vi "Check wait.vi"(11 "Trigger":refnum<vi>) -> (3 "Wait done?":bool)   [LabVIEW 2016]
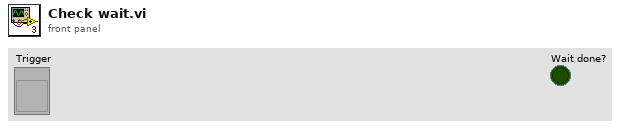
[diagram p1: front panel]
types:
  T1 = typedef "Test settings.ctl" = cluster{"Speed (mm/s)":dbl, "Position limit":bool, "Position limit (mm)":dbl, "Load limit":bool, "Load limit (N)":dbl, "No. of repeats":u16, "Test identifier":string, "Time wait":bool, "Wait time (s)":dbl, "Trigger wait":bool, "Send trigger":bool, "Test notes":string, "Snap intervals":bool, "Time interval (s)":dbl}
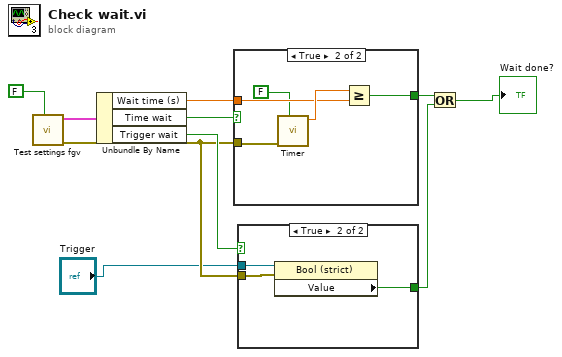
[diagram p0: block diagram]
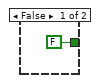
[diagram p2: hidden frame]
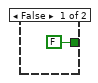
[diagram p3: hidden frame]
diagram:
  n1 = call "Test settings fgv.vi"("Set?"=FALSE) -> ("error out"=w2:errorcluster, "Test settings out"=w9:T1)  [unwired: 8 in, 1 out]
  n2 = Unbundle By Name(w9) -> ("Wait time (s)"=w7:dbl, "Time wait"=w8:bool, "Trigger wait"=w6:bool)
  n3 = case shown="True" w8 {
    tunnel: w2 -> [_ w16]
    tunnel: w7 -> [_ w14]
    tunnel: [FALSE w13] -> w5
    frame False {
    }
    frame True {
      n4 = call "Timer.vi"("Reset"=FALSE, "error in (no error)"=w16) -> ("Time (s)"=w15:dbl)  [unwired: 8 in, 1 out]
      n5 = Greater Or Equal?(x=w15, y=w14) -> (x >= y?=w13:bool)
    }
  }
  n6 = case shown="True" w6 {
    tunnel: "Trigger" -> [_ w20]
    tunnel: [FALSE ("Value") w19] -> w4
    tunnel: w2 -> [_ w18]
    frame False {
    }
    frame True {
      n7 = property class="Bool (strict)"(reference=w20, error in=w18) -> ("Value"=w19:bool)  [unwired: 2 out]
    }
  }
  n8 = Or(x=w5, y=w4) -> (x .or. y?=→"Wait done?":bool)
